vi "scripting_v2.vi"() -> ()   [LabVIEW 2020]
uses:
  <vilib>/numeric/LVNumericRepresentation.ctl
panel:
  out "appended path":path
  out "concatenated string":string
  out "resulting string":string
  out "error out 2":errorcluster
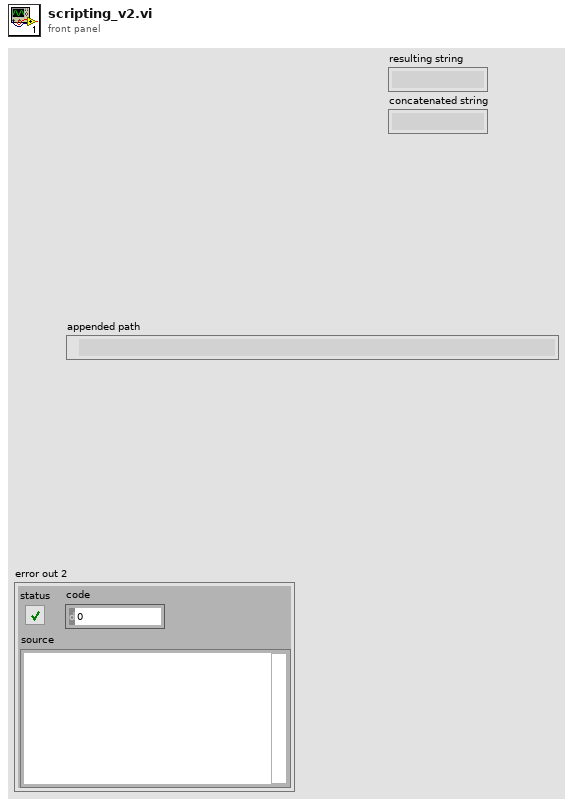
[diagram p1: front panel]
types:
  T1 = typedef "LVNumericRepresentation.ctl" = enum32{"Extended Precision", "Double Precision", "Single Precision", "Long", "Word", "Byte", "Unsigned Long", "Unsigned Word", "Unsigned Byte", "Complex Extended", "Complex Double", "Complex Single", "Quad", "Unsigned Quad", "Fixed-Point"}
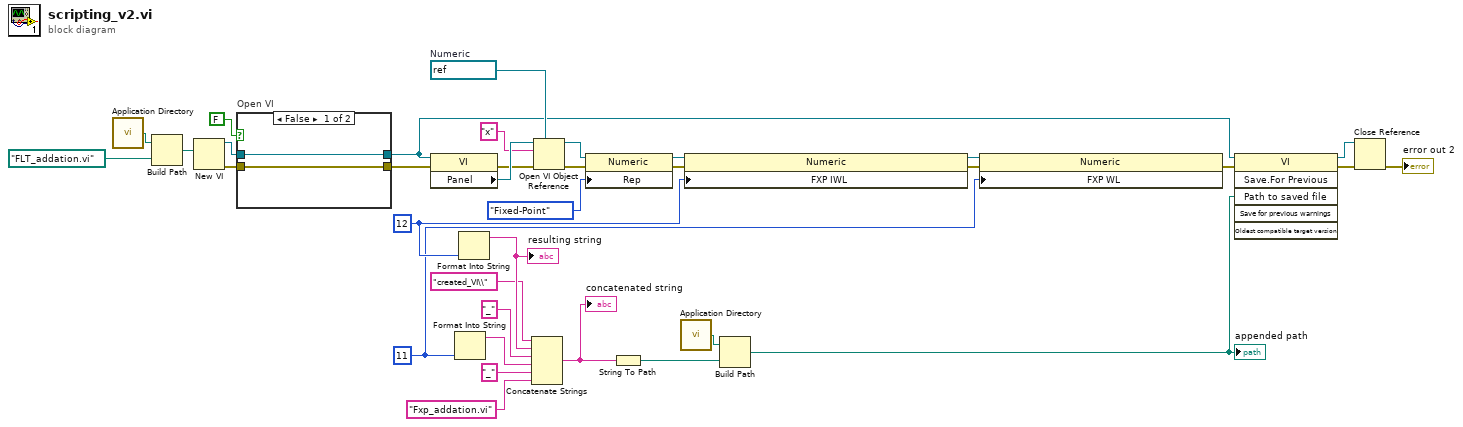
[diagram p0: block diagram]
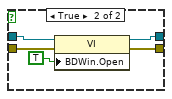
[diagram p2: hidden frame]
diagram:
  w7 = 11 ("Fixed-Point Representation:Bits:Word Length")
  w10 = 12 ("Fixed-Point Representation:Bits:Integer Word Length")
  w29 = refnum<vi> refnum  # Numeric
  n1 = call <vilib>:"Application Directory.vi"() -> ("Application Directory"=w15:path)
  n2 = Build Path(base path=w15, name or relative path=path "FLT_addation.vi" ("vi path")) -> (appended path=w13:path)
  n3 = New VI(10:w13) -> (0:w34:errorcluster, 3:w35:refnum<vi>)  [unwired: 6 in]
  n4 = case "Open VI" shown="False" FALSE {
    tunnel: w35 -> [w36 w42]
    tunnel: w34 -> [w37 w41]
    tunnel: [w36 w39] -> w21
    tunnel: [w37 w38] -> w22
    frame False {
    }
    frame True {
      n5 = property class="VI"(reference=w42, error in=w41, "BDWin.Open"=TRUE ("Block Diagram Window:Open")) -> (reference out=w39:refnum<vi>, error out=w38:errorcluster)
    }
  }
  n6 = property on="Property Node" class="VI"(reference=w21, error in=w22) -> (error out=w25:errorcluster, "Panel"=w27:refnum<vi>)  [unwired: 1 out]
  n7 = Format Into String(w7) -> (resulting string=w6:string)  [unwired: 3 in, 1 out]
  n8 = Format Into String(w10) -> (resulting string=w9:string)  [unwired: 3 in, 1 out]
  "resulting string" <- w9
  n9 = Concatenate Strings("created_VI\\" ("string"), w9, "_" ("string"), w6, "_" ("string"), "Fxp_addation.vi" ("string")) -> (w4:string)
  "concatenated string" <- w4
  n10 = Open VI Object Reference(7:w29, 8:w25, 10:"x" ("name/order"), 11:w27) -> (0:w26:errorcluster, 3:w28:refnum<vi>)
  n11 = property on="Property Node" class="Numeric"(reference=w28, error in=w26, "Rep"=LVNumericRepresentation."Fixed-Point" ("new representation")) -> (reference out=w20:refnum<vi>, error out=w19:errorcluster)
  n12 = String To Path(string=w4) -> (path=w2:path)
  n13 = call <vilib>:"Application Directory.vi"() -> ("Application Directory"=w12:path)
  n14 = property on="Property Node" class="Numeric"(reference=w20, error in=w19, "FXP IWL"=w10) -> (reference out=w18:refnum<vi>, error out=w17:errorcluster)
  n15 = Build Path(base path=w12, name or relative path=w2) -> (appended path=w11:path)
  "appended path" <- w11
  n16 = property on="Property Node" class="Numeric"(reference=w18, error in=w17, "FXP WL"=w7) -> (error out=w16:errorcluster)  [unwired: 1 out]
  n17 = invoke class="VI" method="Save.For Previous"(reference=w21, error in=w16, "Path to saved file"=w11) -> (reference out=w33:refnum<vi>, error out=w32:errorcluster)  [unwired: 3 in, 4 out]
  n18 = Close Reference(reference=w33, error in (no error)=w32) -> (error out=→"error out 2":errorcluster)
